vi "Get SMO Name.vi"(8 "error in (no error)":errorcluster, 11 "Example Instrument in":refnum<class "Instrument.LN2.lvclass">) -> (0 "error out":errorcluster, 2 "SMO Name":string, 3 "Example Instrument out":refnum<class "Instrument.LN2.lvclass">)   [LabVIEW 2019, in "Instrument.LN2.lvclass"]
uses:
  Instrument.LN2.lvclass
  <userlib>/LevyLab/Instrument Framework/Instrument Types/VSource/Instrument.VSource.lvclass
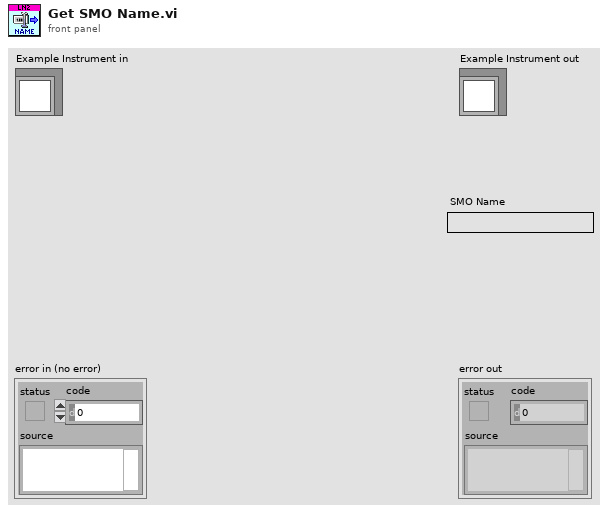
[diagram p1: front panel]
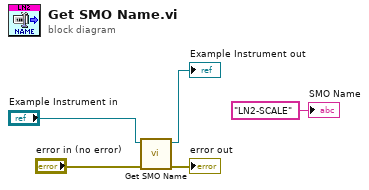
[diagram p0: block diagram]
diagram:
  n1 = call-parent "Get SMO Name.vi"("error in (no error)"="error in (no error)", "Instrument in"="Example Instrument in") -> ("error out"=→"error out":errorcluster, "Instrument out"=→"Example Instrument out":refnum<class "Instrument.LN2.lvclass">)  [unwired: 7 in, 1 out]
  "SMO Name" <- "LN2-SCALE" ("SMO Name")
